vi "Read stage name and version.vi"(8 "error in (no error)":errorcluster, 11 "_stage in":refnum<class "_stage.lvclass">) -> (0 "error out":errorcluster, 2 "stage name and version":string, 3 "_stage out":refnum<class "_stage.lvclass">)   [LabVIEW 2019, in "_stage.lvlib" / "_stage.lvclass"]
uses:
  _stage.lvclass
  _stage.lvclass/_stage.ctl
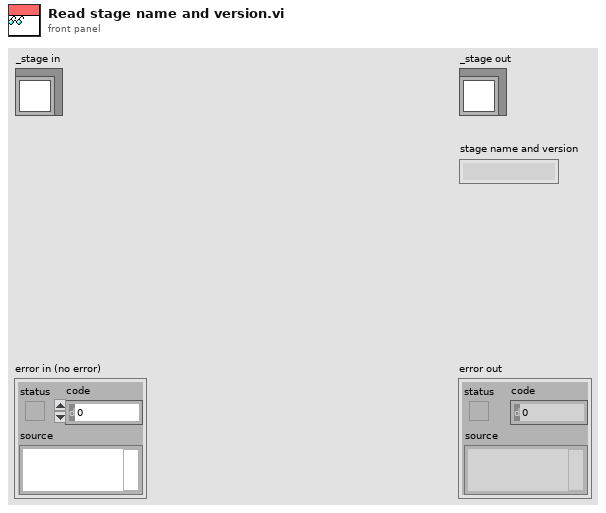
[diagram p1: front panel]
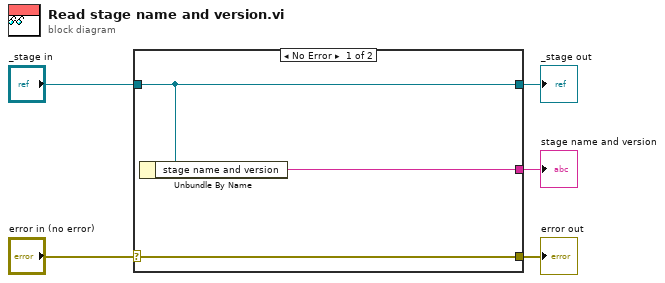
[diagram p0: block diagram]
diagram:
  n1 = case shown="No Error" "error in (no error)" {
    selector: "error in (no error)" -> [w8 w9]
    tunnel: [w8 w9] -> w4
    tunnel: [w7 w10] -> w2
    tunnel: "_stage in" -> [w7 w10]
    tunnel: [w6 _] -> w1
    frame No Error {
      n2 = Unbundle By Name(w7) -> ("stage name and version"=w6:string)
    }
    frame Error {
    }
  }
  "error out" <- w4
  "_stage out" <- w2
  "stage name and version" <- w1
